vi "Process Thread.vi"(8 "error in (no error)":errorcluster) -> (0 "error out":errorcluster)   [LabVIEW 2020]
doc: "Process thread is used for all internal process"
uses:
  FGV/Controls/FGV_State.ctl
  Controls/Data_Initialize.ctl
  Database/Controls/Account Database.ctl
  Controls/Events_User.ctl
  Database/Controls/Todo.ctl
  SubVIs/Message Queue/Enqueue Message (Single).vi
  <vilib>/Utility/error.llb/Error Cluster From Error Code.vi
  <vilib>/ErrorRing/Error Ring.xnode
  SubVIs/Message Queue/Message Queue.lvlib
types:
  T1 = enum32{"Invalid", "Standard", "Closed", "Hidden", "Minimized", "Maximized"}
  T2 = typedef "FGV_State.ctl" = enum16{"1 - OpenDatabase", "2 - Initialize Events", "3 - Initialize QMH", "4 - Close QMH", "5 - Close Events", "Read FGV", "Save Database", "Def"}
  T3 = typedef "FGV_Data.ctl" = cluster{"QMH":T4, "User Events":T5, "Database":T6[]}
  T4 = typedef "Message Queue.lvlib/All Message Queues.ctl" = cluster{"User Console":refnum<queue>, "Display Console":refnum<queue>, "Sensor Interface":refnum<queue>, "Process":refnum<queue>}
  T5 = typedef "Events_User.ctl" = cluster{"Stop User Console":refnum<user-event>, "Error User Console":refnum<user-event>, "Stop Sensor Interface ":refnum<user-event>, "Error Sensor Interface":refnum<user-event>}
  T6 = typedef "Account Database.ctl" = cluster{"Account Number":i32, "First Name":string, "Last Name":string, "Balance":dbl}
  T7 = typedef "Data_Initialize.ctl" = cluster{"Database":T6[], "User Events":T5}
  T8 = typedef "Todo.ctl" = enum16{"Read", "Update"}
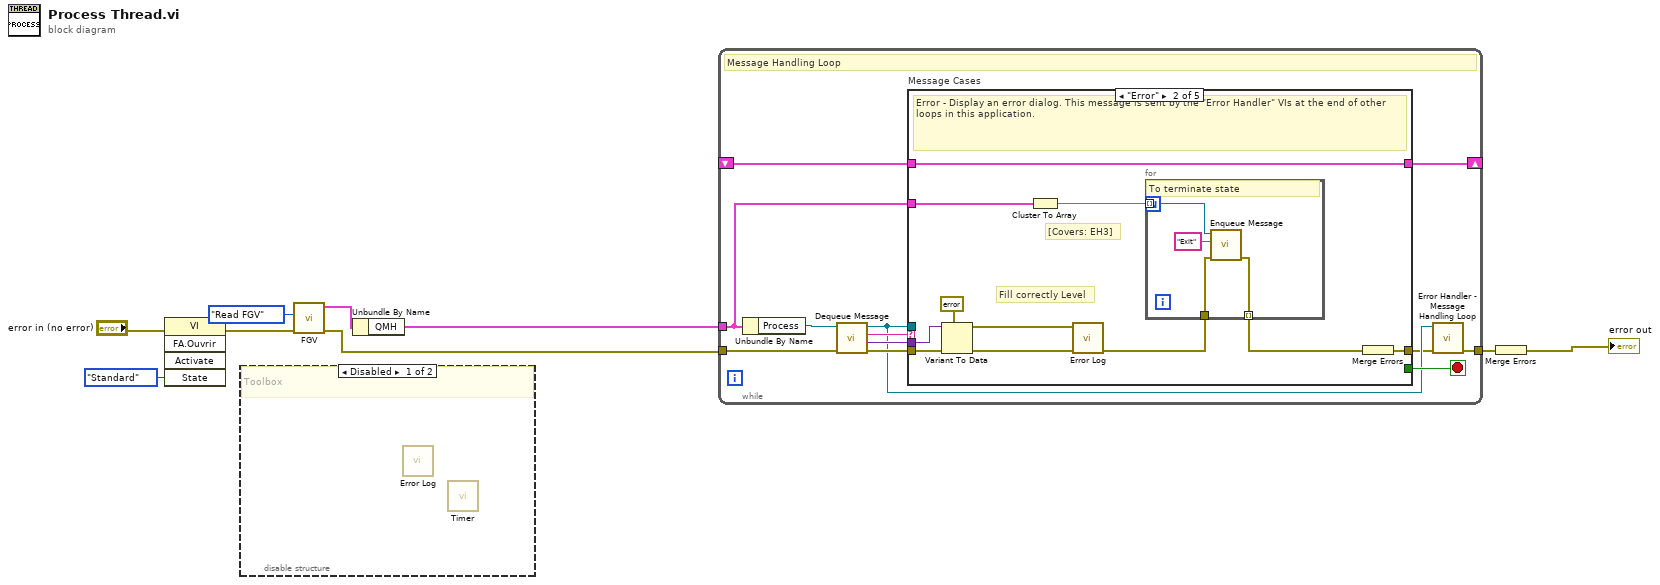
[diagram p0: block diagram]
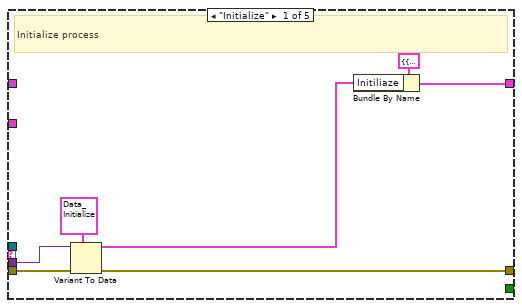
[diagram p3: hidden frame]
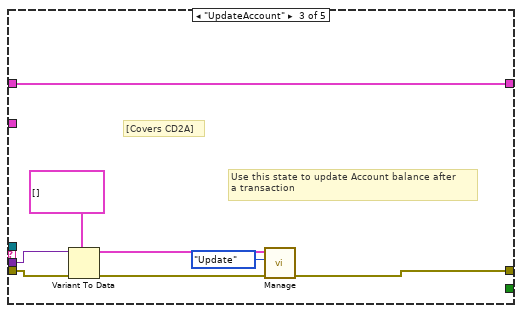
[diagram p4: hidden frame]
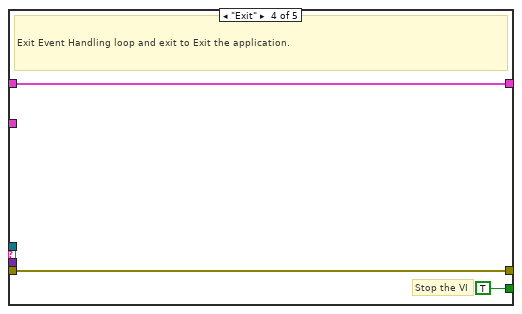
[diagram p5: hidden frame]
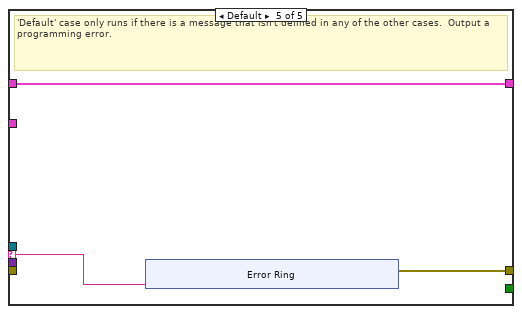
[diagram p6: hidden frame]
diagram:
  n1 = invoke class="VI" method="FA.Ouvrir"(error in="error in (no error)", "State"=T1."Standard") -> (error out=w3:errorcluster)  [unwired: 3 in, 4 out]
  n2 = disable-structure shown="Disabled" {
    frame Disabled {
      # "Toolbox"
      n3 = call "Error Log.vi"() -> ()  [unwired: 11 in, 1 out]
      n4 = call "Timer.vi"() -> ()  [unwired: 9 in, 3 out]
    }
    frame Enabled {
    }
  }
  n5 = call "FGV.vi"("error in (no error)"=w3, "FGV_State"=FGV_State."Read FGV") -> ("error out"=w1:errorcluster, "FGV"=w7:T3)  [unwired: 8 in]
  n6 = Unbundle By Name(w7) -> ("QMH"=w9:T4)
  n7 = while {
    tunnel: w9 -> [w10]
    shift-right: [w20] -> _
    shift-left: _ -> [w21]
    tunnel: w1 -> [w18]
    tunnel: [w13] -> w5
    stop <- w19 stop-if-true
    # "Message Handling Loop"
    n8 = Unbundle By Name(w10) -> ("Process"=w11:refnum<queue>)
    n9 = call "Dequeue Message.vi"("error in (no error)"=w18, "Message Queue"=w11) -> ("error out"=w17:errorcluster, "Message Data"=w15:variant, "Message"=w16:string, "dup Message Queue"=w14:refnum<queue>)  [unwired: 6 in]
    n10 = case "Message Cases" shown="\"Error\"" w16 {
      selector: w16 -> [_ _ _ _ w55]
      tunnel: w14 -> [_ _ _ _ _]
      tunnel: w17 -> [w26 w39 w50 w52 _]
      tunnel: [w23 w36 w46 w52 w56] -> w12
      tunnel: w21 -> [_ w33 w51 w53 w57]
      tunnel: [w28 w33 w51 w53 w57] -> w20
      tunnel: [_ _ _ TRUE _] -> w19
      tunnel: w15 -> [w22 w38 w49 _ _]
      tunnel: w10 -> [_ w32 _ _ _]
      frame "Initialize" {
        # "Initialize process"
        n11 = Variant To Data(error in=w26, type=T7 {"Database"=[], "User Events"={"Stop User Console"=refnum, "Error User Console"=refnum, "Stop Sensor Interface "=refnum, "Error Sensor Interface"=refnum}} ("Initiliaze"), Variant=w22) -> (data=w24:T7, error out=w23:errorcluster)
        n12 = Bundle By Name(cluster=cluster{"Initiliaze":T7} {"Initiliaze"={"Database"=[], "User Events"={"Stop User Console"=refnum, "Error User Console"=refnum, "Stop Sensor Interface "=refnum, "Error Sensor Interface"=refnum}}} ("Local Data"), "Initiliaze"=w24) -> (w28:cluster{"Initiliaze":T7})
      }
      frame "Error" {
        # "[Covers: EH3]"
        # "Fill correctly Level"
        # "Error - Display an error dialog. This message is sent by the \"Error Handler\" VIs at the end of other loops in this application."
        n13 = Variant To Data(error in=w39, type=errorcluster {"status"=FALSE, "code"=0, "source"=""} ("error constant"), Variant=w38) -> (data=w34:errorcluster, error out=w35:errorcluster)
        n14 = Cluster To Array(cluster=w32) -> (array=w31:refnum<queue>[])
        n15 = call "Error Log.vi"("error in"=w35, "error happened"=w34) -> ("error out"=w30:errorcluster)  [unwired: 9 in]
        n16 = for {
          tunnel: w31 -> [w43] mode=indexing
          tunnel: w30 -> [w42]
          tunnel: [w41] -> w29 mode=indexing
          # "To terminate state"
          n17 = call-poly "Enqueue Message.vi"("error in (no error)"=w42, "Message"="Exit", "Message Queue"=w43) -> ("error out"=w41:errorcluster)  [unwired: 7 in, 1 out]
        }
        n18 = Merge Errors(w29) -> (w36:errorcluster)
      }
      frame "UpdateAccount" {
        # "Use this state to update Account balance after \na transaction"
        # "[Covers CD2A]"
        n19 = Variant To Data(error in=w50, type=T6[] [] ("Database IN"), Variant=w49) -> (data=w45:T6[], error out=w47:errorcluster)
        n20 = call "Manage.vi"("error in"=w47, "ToDo"=Todo."Update", "Database IN"=w45) -> ("error out"=w46:errorcluster)  [unwired: 7 in, 1 out]
      }
      frame "Exit" {
        # "Stop the VI"
        # "Exit Event Handling loop and exit to Exit the application."
      }
      frame Default {
        # "'Default' case only runs if there is a message that isn't defined in any of the other cases.  Output a programming error."
        n21 = xnode "Error Ring"("paramètre 0"=w55) -> ("sortie d'erreur"=w56:errorcluster)
      }
    }
    n22 = call "Error Handler - Message Handling Loop.vi"("error in (no error)"=w12, "Message Queue"=w14) -> ("dup error in"=w13:errorcluster)  [unwired: 8 in, 1 out]
  }
  n23 = Merge Errors(w5) -> (→"error out":errorcluster)
